vi "4_3.vi"() -> ()   [LabVIEW 2020]
uses:
  <vilib>/numeric/Random Number (Range) U64.vi
  <vilib>/numeric/sub_Random U32.vi
panel:
  out "Array Output":dbl[](array[numeric])
  out "Array 2":dbl[](array[numeric])
  out "Array":dbl[](array[numeric])
  in  "Size 2":dbl
  in  "Size 1":dbl
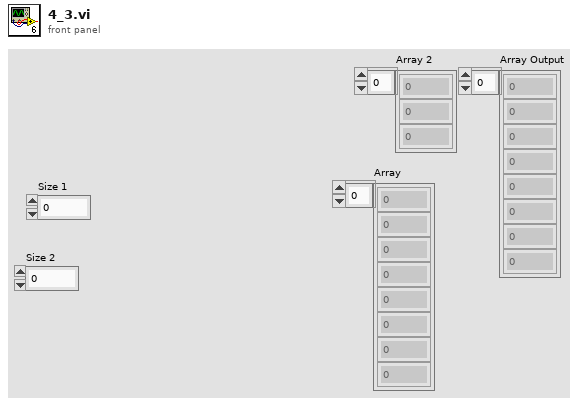
[diagram p1: front panel]
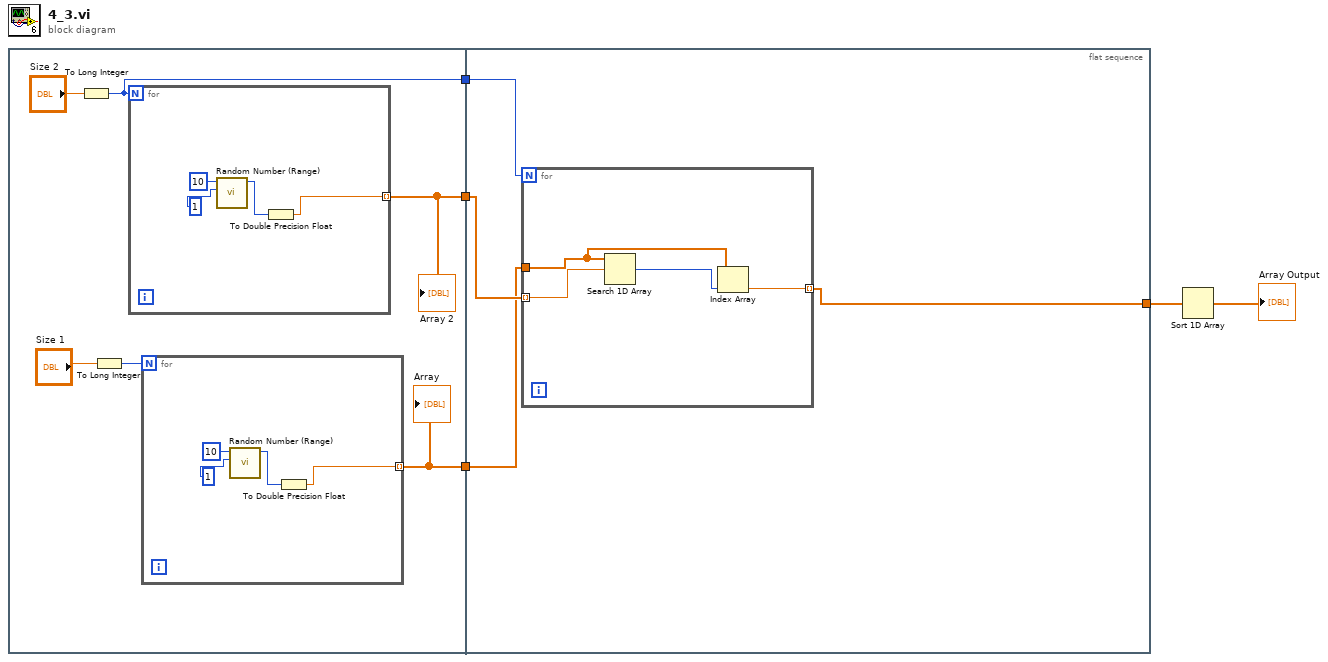
[diagram p0: block diagram]
diagram:
  n1 = flat-sequence {
    tunnel: [w8] -> w5
    tunnel: [w7] -> w4
    tunnel: [w6] -> w3
    tunnel: w5 -> [w23]
    tunnel: w4 -> [w22]
    tunnel: w3 -> [w21]
    tunnel: [w20] -> w1
    frame #0 {
      n2 = To Long Integer(number="Size 2") -> (32bit integer=w8:i32)
      n3 = To Long Integer(number="Size 1") -> (32bit integer=w10:i32)
      n4 = for {
        N: w8 -> [_]
        tunnel: [w16] -> w7 mode=indexing
        n5 = call-poly <vilib>:"Random Number (Range).vi"("lower bound (0)"=u64 1 ("upper bound (100)"), "upper bound (100)"=u64 10) -> ("number"=w17:u64)  [unwired: 9 in]
        n6 = To Double Precision Float(number=w17) -> (double precision float=w16:dbl)
      }
      "Array 2" <- w7
      n7 = for {
        N: w10 -> [_]
        tunnel: [w12] -> w6 mode=indexing
        n8 = call-poly <vilib>:"Random Number (Range).vi"("lower bound (0)"=u64 1 ("upper bound (100)"), "upper bound (100)"=u64 10) -> ("number"=w13:u64)  [unwired: 9 in]
        n9 = To Double Precision Float(number=w13) -> (double precision float=w12:dbl)
      }
      "Array" <- w6
    }
    frame #1 {
      n10 = for {
        N: w23 -> [_]
        tunnel: [w26] -> w20 mode=indexing
        tunnel: w21 -> [w25]
        tunnel: w22 -> [w24] mode=indexing
        n11 = Search 1D Array(1D array=w25, element=w24) -> (index of element=w27:i32)  [unwired: 1 in]
        n12 = Index Array(array=w25, index=w27) -> (element=w26:dbl)
      }
    }
  }
  n13 = Sort 1D Array(array=w1) -> (sorted array=→"Array Output":dbl[])
